vi "Periodic Tasks.vi"(8 "error in":errorcluster) -> ()   [LabVIEW 2017]
doc: "This VI runs in parallel to other tasks. It can contain as many user-defined periodic loops as you need. These can carry out PID or other sorts of timed response."
uses:
  <vilib>/Rock Robotics/WPI/DriverStation/WPI_DriverStationRobotMode2.ctl
  <vilib>/Rock Robotics/WPI/Utilities/WPI_GetSetVariantRefNum.vi
  <vilib>/Rock Robotics/Network Tables/NT Write Numeric Array.vi
  <vilib>/Rock Robotics/Network Tables/NT Write Boolean Array.vi
  <vilib>/Rock Robotics/Network Tables/NT Write Number.vi
  <vilib>/Rock Robotics/WPI/RobotDrive/WPI_RobotDriveArcadeDrive_Standard(NoSaturation).vi
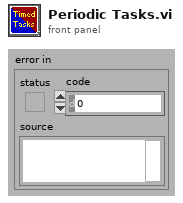
[diagram p1: front panel]
types:
  T1 = typedef "WPI_DriverStationRobotMode2.ctl" = enum16{"Autonomous Disabled", "Autonomous Enabled", "Teleop Disabled", "Teleop Enabled", "Disconnected", "Finish", "Test Disabled", "Test Enabled", "Emergency Stopped"}
  T2 = typedef "WPI_JoystickDevRef.ctl" = cluster{"Device":T3}
  T3 = typedef "WPI_JoystickDeviceEnum.ctl" = enum16{"USB 0", "USB 1", "USB 2", "USB 3", "USB 4", "USB 5"}
  T4 = typedef "WPI_GyroDevRef.ctl" = cluster{"DevStatus":errorcluster, "Analog Channel":T5, "Gain (VoltsPerDegree/Second)":dbl, "Gyro Type":enum16{"Analog", "XRS450"}, "Handle":i32, "SPI Bus":T6, "Device Found":bool, "Sample Rate":dbl, "Calibrate On Open":bool, "Offset":dbl}
  T5 = typedef "FPGA_AIChannel.ctl" = enum8{"AI 0", "AI 1", "AI 2", "AI 3", "AI MXP 0", "AI MXP 1", "AI MXP 2", "AI MXP 3", "Invalid"}
  T6 = typedef "spi_bus.ctl" = enum16{"SPI On-Board, CS0", "SPI On-Board, CS1", "SPI On-Board, CS2", "SPI On-Board, CS3", "SPI MXP", "Invalid"}
  T7 = typedef "WPI_RobotDriveDevRef.ctl" = cluster{"DevStatus":errorcluster, "Motors[]":T8[], "Square Inputs":bool, "Max Output":dbl}
  T8 = typedef "WPI_MotorControlDeviceRef.ctl" = cluster{"DeviceStatus":errorcluster, "Type":T9, "PWM":cluster{"PWM Channel":T10, "DeadBand":T11}, "CAN":cluster{"Device Number":u8, "SetOutput VI Ref":variant, "GetOutput VI Ref":variant, "Enable VI Ref":variant, "Disable VI Ref":variant, "Data":variant}, "Invert":bool, "DIO PWM":cluster{"PWM \"Enable\" Channel":T10, "DIOChannel":T12, "PWM Rate":dbl}}
  T9 = typedef "WPI_MotorControlType.ctl" = enum16{"PWM", "CAN", "DIO PWM"}
  T10 = typedef "FPGA_DIOPWMChannel.ctl" = enum8{"PWM 0", "PWM 1", "PWM 2", "PWM 3", "PWM 4", "PWM 5", "PWM 6", "PWM 7", "PWM 8", "PWM 9", "PWM MXP 0", "PWM MXP 1", "PWM MXP 2", "PWM MXP 3", "PWM MXP 4", "PWM MXP 5", "PWM MXP 6", "PWM MXP 7", "PWM MXP 8", "PWM MXP 9", "Invalid"}
  T11 = typedef "WPI_PWMDeadband.ctl" = cluster{"Name":string, "maxPositivePwm":i32, "minPositivePwm":i32, "centerPwm":i32, "maxNegativePwm":i32, "minNegativePwm":i32, "angularRange":u16}
  T12 = typedef "FPGA_DIOChannel.ctl" = enum8{"DIO 0", "DIO 1", "DIO 2", "DIO 3", "DIO 4", "DIO 5", "DIO 6", "DIO 7", "DIO 8", "DIO 9", "DIO MXP 0", "DIO MXP 1", "DIO MXP 2", "DIO MXP 3", "DIO MXP 4", "DIO MXP 5", "DIO MXP 6", "DIO MXP 7", "DIO MXP 8", "DIO MXP 9", "DIO MXP 10", "DIO MXP 11", "DIO MXP 12", "DIO MXP 13", "DIO MXP 14", "DIO MXP 15", "SPI Port CS1", "SPI Port CS2", "SPI Port CS3", "SPI Port MISO", "SPI Port MOSI", "Invalid"}
  T13 = cluster{"JoystickDevRef":T2, "RobotDriveDevRef":T7}
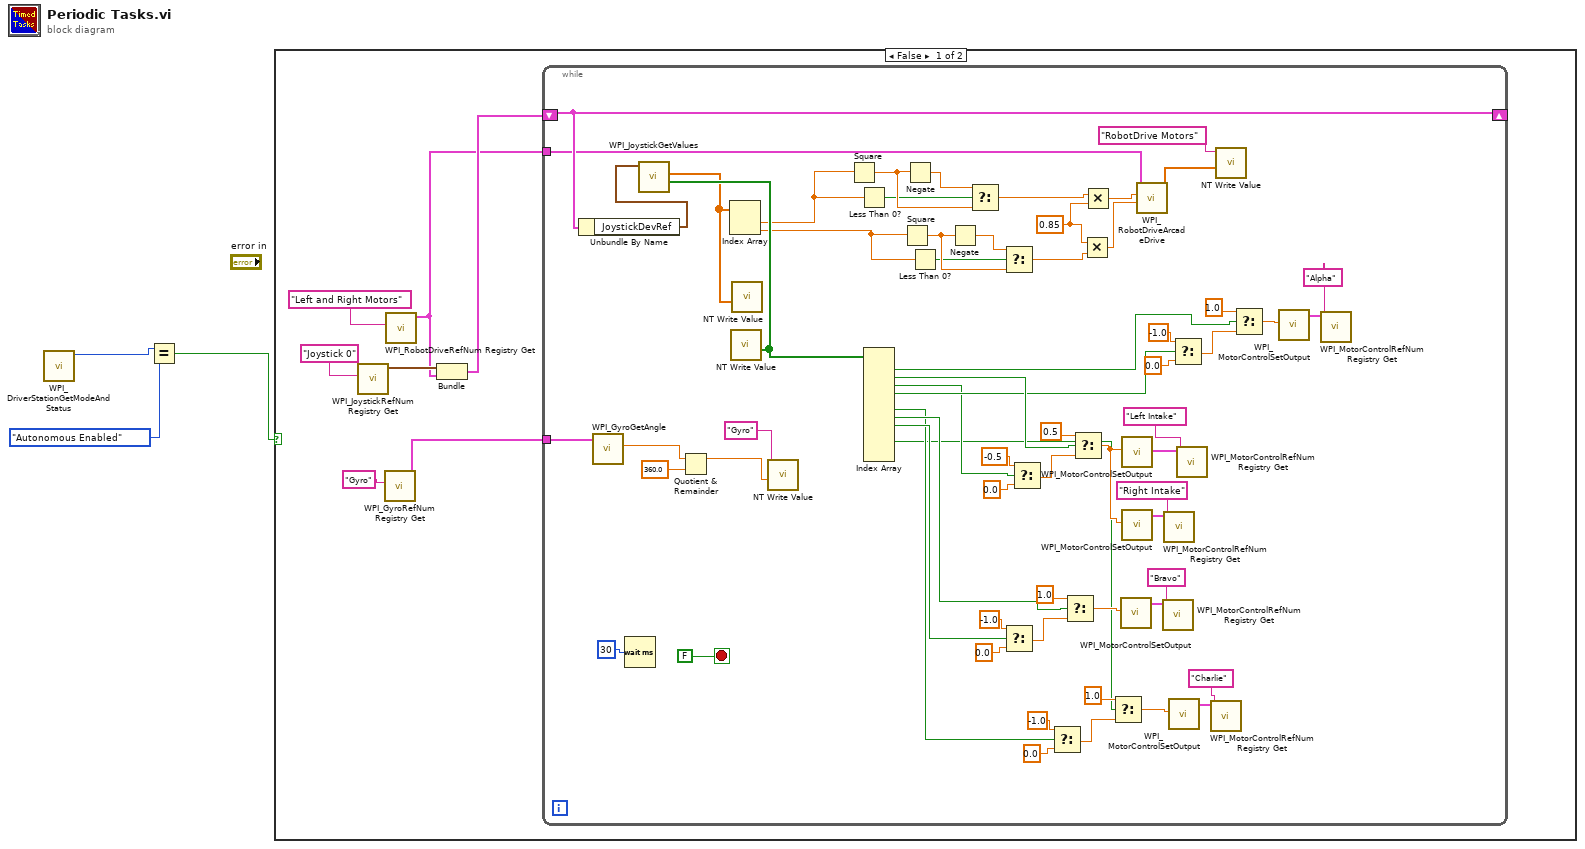
[diagram p0: block diagram]
diagram:
  n1 = call <vilib>:"WPI_DriverStationGetModeAndStatus.vi"() -> ("Robot Mode"=w3:T1)  [unwired: 10 in, 1 out]
  n2 = Equal?(x=w3, y=WPI_DriverStationRobotMode2."Autonomous Enabled") -> (x = y?=w1:bool)
  n3 = case shown="False" w1 {
    frame False {
      n4 = call <vilib>:"WPI_JoystickRefNum Registry Get.vi"("refnum name"="Joystick 0") -> ("JoystickDevRef"=w8:T2)  [unwired: 1 in, 9 out]
      n5 = call <vilib>:"WPI_GyroRefNum Registry Get.vi"("refnum name"="Gyro") -> ("GyroDevRef"=w5:T4)  [unwired: 9 in, 1 out]
      n6 = call <vilib>:"WPI_RobotDriveRefNum Registry Get.vi"("refnum name"="Left and Right Motors") -> ("RobotDriveDevRef"=w6:T7)  [unwired: 1 in, 9 out]
      n7 = Bundle("JoystickDevRef"=w8, "RobotDriveDevRef"=w6) -> (w7:T13)  [unwired: 1 out]
      n8 = while {
        shift-right: [w66] -> _
        shift-left: w7 -> [w66]
        tunnel: w6 -> [w42]
        tunnel: w5 -> [w52]
        stop <- FALSE stop-if-true
        w12 = 0.85 ("x*y")
        n9 = Unbundle By Name(w66) -> ("JoystickDevRef"=w67:T2)
        n10 = call <vilib>:"WPI_GyroGetAngle.vi"("GyroDevRef"=w52) -> ("Angle"=w50:dbl)  [unwired: 6 in, 4 out]
        n11 = Wait (ms)(milliseconds to wait=u32 30) -> ()  [unwired: 1 out]
        n12 = call <vilib>:"WPI_JoystickGetValues.vi"("JoystickDevRef"=w67) -> ("Buttons"=w71:bool[], "Axes"=w68:dbl[])  [unwired: 6 in, 3 out]
        n13 = Quotient & Remainder(x=w50, y=360.0) -> (x-y*floor(x/y)=w49:dbl)  [unwired: 1 out]
        n14 = Index Array(array=w68) -> (element #1=w57:dbl, element #2=w53:dbl)  [unwired: 2 in]
        n15 = call-poly <vilib>:"NT Write Value.vi"("Boolean Array"=w71) -> ()  [unwired: 10 in, 1 out]
        n16 = call-poly <vilib>:"NT Write Value.vi"("Numeric Array"=w68) -> ()  [unwired: 10 in, 1 out]
        n17 = call-poly <vilib>:"NT Write Value.vi"("Numeric"=w49, "Name"="Gyro") -> ()  [unwired: 9 in, 1 out]
        n18 = Square(x=w57) -> (x^2=w60:dbl)
        n19 = Less Than 0?(x=w57) -> (x < 0?=w58:bool)
        n20 = Index Array(array=w71) -> (element #1=w61:bool, element #2=w36:bool, element #3=w34:bool, element #4=w35:bool, element #6=w17:bool, element #7=w26:bool, element #8=w25:bool, element #10=w16:bool)  [unwired: 12 in, 4 out]
        n21 = Square(x=w53) -> (x^2=w56:dbl)
        n22 = Negate(x=w60) -> (-x=w59:dbl)
        n23 = Less Than 0?(x=w53) -> (x < 0?=w54:bool)
        n24 = Negate(x=w56) -> (-x=w55:dbl)
        n25 = Select(t=w59, s=w58, f=w60) -> (s? t:f=w15:dbl)
        n26 = Select(t=w55, s=w54, f=w56) -> (s? t:f=w13:dbl)
        n27 = Select(t=-1.0, s=w25, f=0.0) -> (s? t:f=w28:dbl)
        n28 = Select(t=-0.5, s=w34, f=0.0) -> (s? t:f=w43:dbl)
        n29 = Select(t=-1.0, s=w17, f=0.0) -> (s? t:f=w19:dbl)
        n30 = Select(t=1.0, s=w26, f=w28) -> (s? t:f=w27:dbl)
        n31 = Select(t=0.5, s=w36, f=w43) -> (s? t:f=w37:dbl)
        n32 = Multiply(x=w12, y=w13) -> (x*y=w11:dbl)
        n33 = Multiply(x=w15, y=w12) -> (x*y=w14:dbl)
        n34 = Select(t=1.0, s=w16, f=w19) -> (s? t:f=w18:dbl)
        n35 = call-poly <vilib>:"WPI_RobotDriveArcadeDrive.vi"("Y axis value"=w11, "X axis value"=w14, "RobotDriveDevRef"=w42) -> ("Motor Values"=w73:dbl[])  [unwired: 6 in, 2 out]
        n36 = call <vilib>:"WPI_MotorControlRefNum Registry Get.vi"("refnum name"="Bravo") -> ("MotorControlDevRef"=w32:T8)  [unwired: 9 in, 1 out]
        n37 = call <vilib>:"WPI_MotorControlSetOutput.vi"("Output"=w27, "MotorControlDevRef"=w32) -> ()  [unwired: 7 in, 3 out]
        n38 = call <vilib>:"WPI_MotorControlRefNum Registry Get.vi"("refnum name"="Right Intake") -> ("MotorControlDevRef"=w39:T8)  [unwired: 9 in, 1 out]
        n39 = call <vilib>:"WPI_MotorControlSetOutput.vi"("Output"=w37, "MotorControlDevRef"=w39) -> ()  [unwired: 7 in, 3 out]
        n40 = Select(t=-1.0, s=w35, f=0.0) -> (s? t:f=w62:dbl)
        n41 = call <vilib>:"WPI_MotorControlRefNum Registry Get.vi"("refnum name"="Left Intake") -> ("MotorControlDevRef"=w41:T8)  [unwired: 9 in, 1 out]
        n42 = call <vilib>:"WPI_MotorControlSetOutput.vi"("Output"=w37, "MotorControlDevRef"=w41) -> ()  [unwired: 7 in, 3 out]
        n43 = call <vilib>:"WPI_MotorControlRefNum Registry Get.vi"("refnum name"="Charlie") -> ("MotorControlDevRef"=w23:T8)  [unwired: 9 in, 1 out]
        n44 = call <vilib>:"WPI_MotorControlSetOutput.vi"("Output"=w18, "MotorControlDevRef"=w23) -> ()  [unwired: 7 in, 3 out]
        n45 = call-poly <vilib>:"NT Write Value.vi"("Numeric Array"=w73, "Name"="RobotDrive Motors") -> ()  [unwired: 9 in, 1 out]
        n46 = Select(t=1.0, s=w61, f=w62) -> (s? t:f=w33:dbl)
        n47 = call <vilib>:"WPI_MotorControlRefNum Registry Get.vi"("refnum name"="Alpha") -> ("MotorControlDevRef"=w70:T8)  [unwired: 9 in, 1 out]
        n48 = call <vilib>:"WPI_MotorControlSetOutput.vi"("Output"=w33, "MotorControlDevRef"=w70) -> ()  [unwired: 7 in, 3 out]
      }
    }
    frame True {
    }
  }
